vi "Enable Disable UI.vi"(8 "error in (no error)":errorcluster, 10 "Disable?":bool, 11 "Reference Array in":refnum<vi>[](array[refnum])) -> (0 "error out":errorcluster, 3 "Reference Array out":refnum<vi>[](array[refnum]))   [LabVIEW 2012, in "Image UDP Broadcast Custom Device.lvlib"]
uses:
  Shared/Image UDP Broadcast Custom Device.lvlib
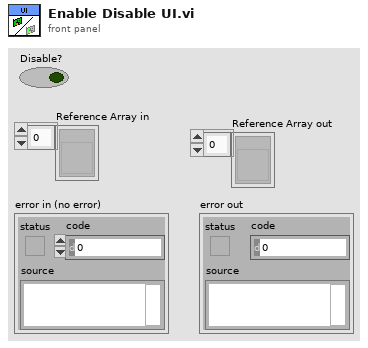
[diagram p1: front panel]
types:
  T1 = enum8{"Enabled", "Disabled", "Disabled and Grayed Out"}
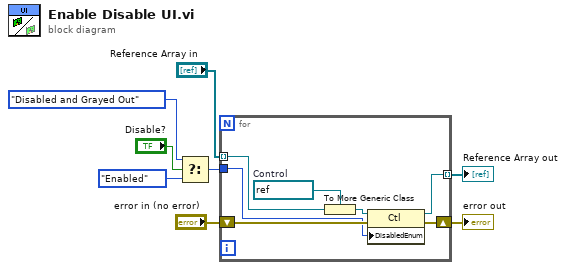
[diagram p0: block diagram]
diagram:
  n1 = Select(t=T1."Disabled and Grayed Out" ("Disabled"), s="Disable?", f=T1."Enabled") -> (s? t:f=w8:T1)
  n2 = for {
    tunnel: "Reference Array in" -> [w15] mode=indexing
    shift-right: [w11] -> w4
    shift-left: "error in (no error)" -> [w12]
    tunnel: w8 -> [w10]
    tunnel: [w9] -> w1 mode=indexing
    w14 = refnum<vi> refnum  # Control
    n3 = To More Generic Class(target class=w14, reference=w15) -> (generic class reference=w13:refnum<vi>)
    n4 = property class="Ctl"(reference=w13, error in=w12, "DisabledEnum"=w10) -> (reference out=w9:refnum<vi>, error out=w11:errorcluster)
  }
  "error out" <- w4
  "Reference Array out" <- w1
